vi "Main.vi"(11 "Module Admin":refnum<class "Delacor_lib_QMH_Module Admin.lvclass">) -> ()   [LabVIEW 2024, in "DAQ.lvlib"]
doc: "This template is based off of the Queued Message Handler design pattern and the Queued Message Handler project template that ships with LabVIEW.\n\nThe main difference is that the queue is private to this module and communication between modules is performed via Broadcast and Request events.\n\nRequest events are wrapped in public API methods and are handled in the Event Handling Loop (EHL) of this VI. Any module can register for Broadcast events sent by this module. The EHL generates messages based on user interface actions.\n\nThe Message Handling Loop (MHL) processes messages generated by the EHL, or by other messages. The messages are string values, so new messages can be added easily to the Message Cases case structure in the MHL. Each message cluster can also provide an optional value for Message Data, which is a variant that can be converted to whatever message-specific data is required.\n_____\nBased on DQMH Project Template 7.0.1.1316."
uses:
  DAQ.lvlib
  <vilib>/Delacor/Delacor QMH/Libraries/Module Admin_class/Delacor_lib_QMH_Module Admin.lvclass
  Module Data--cluster.ctl
  DAQ Config.ctl
  <vilib>/Delacor/Delacor QMH/Libraries/Message Queue_class/Delacor_lib_QMH_Message Queue.lvclass/Delacor_lib_QMH_Message Queue.ctl
  Stop Argument--cluster.ctl
  <vilib>/Delacor/Delacor QMH/Libraries/Module Admin_class/Delacor_lib_QMH_Module Admin.lvclass/Delacor_lib_QMH_Module Admin.ctl
  Configure Acquisition Argument--cluster.ctl
  Start Acquisition Argument--cluster.ctl
  Acquire Argument--cluster.ctl
  Stop Acquisition Argument--cluster.ctl
  <vilib>/Utility/miscctls.llb/LVPointTypeDef.ctl
  <vilib>/Delacor/Delacor QMH/Libraries/Message Queue_class/Delacor_lib_QMH_Enqueue Message (Single).vi
  <vilib>/Delacor/Delacor QMH/Libraries/Module Admin_class/Delacor_lib_QMH_Get External Launch.vi
  <vilib>/DAQmx/create/channels.llb/DAQmx Create Channel (AI-Voltage-Basic).vi
  <vilib>/DAQmx/configure/timing.llb/DAQmx Timing (Sample Clock).vi
  <vilib>/DAQmx/miscellaneous.llb/DAQmx Fill In Error Info.vi
  <vilib>/Delacor/Delacor QMH/Libraries/Message Queue_class/Delacor_lib_QMH_Message Queue.lvclass
  <vilib>/DAQmx/read.llb/DAQmx Read (Analog 1D Wfm NChan NSamp).vi
panel:
  out "Waveform Chart":waveform(dbl)[](graph)
  out "error out":errorcluster
  out "Status":string
  in  "Simulate MHL Error":bool
  in  "Simulate EHL Error":bool
  # "DAQ Module"
  # "This Module runs without a UI"
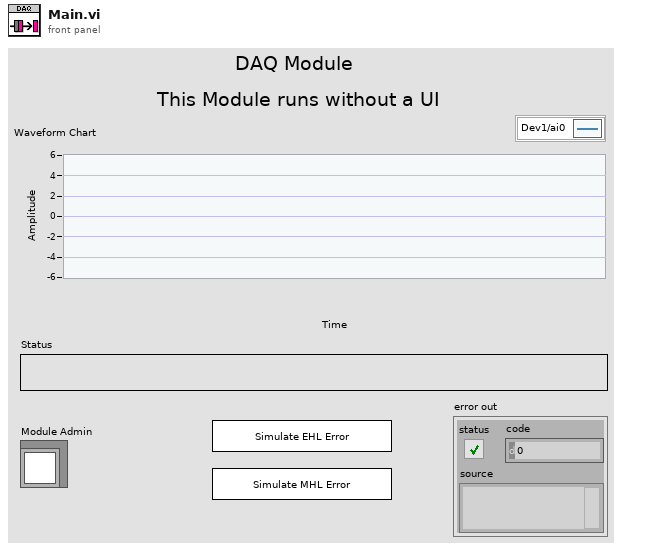
[diagram p1: front panel]
types:
  T1 = typedef "DAQ.lvlib/Request Events--cluster.ctl" = cluster{"Stop Module":refnum<user-event>, "Show Panel":refnum<user-event>, "Hide Panel":refnum<user-event>, "Get Module Execution Status":refnum<user-event>, "Show Diagram":refnum<user-event>, "Configure Acquisition":refnum<user-event>, "Start Acquisition":refnum<user-event>, "Private":cluster{"Acquire":refnum<user-event>}, "Stop Acquisition":refnum<user-event>}
  T2 = typedef "DAQ.lvlib/Module Data--cluster.ctl" = cluster{"Status":string, "DAQ Config":T3, "DAQmx task":refnum<k21>, "Stop Acquisition?":bool}
  T3 = typedef "DAQ.lvlib/DAQ Config.ctl" = cluster{"DAQmx Channel":tag, "Samplerate":dbl, "# Samples":i32}
  T4 = enum32{"invalid lock state", "Not Locked", "Locked (No Password)", "Password-protected"}
  T5 = typedef "DAQ.lvlib/Stop Argument--cluster.ctl" = cluster{"Origin":string, "Exit via Stop Module Req?":bool, "Wait for Module to stop?":bool}
  T6 = typedef "DAQ.lvlib/Configure Acquisition Argument--cluster.ctl" = cluster{"DAQ Config":T3}
  T7 = typedef "DAQ.lvlib/Start Acquisition Argument--cluster.ctl" = cluster{"Boolean":bool}
  T8 = typedef "DAQ.lvlib/Acquire Argument--cluster.ctl" = cluster{"Boolean":bool}
  T9 = typedef "DAQ.lvlib/Stop Acquisition Argument--cluster.ctl" = cluster{"Boolean":bool}
  T10 = typedef "LVPointTypeDef.ctl" = cluster{"Horizontal":i16, "Vertical":i16}
  T11 = enum32{"Invalid", "Standard", "Closed", "Hidden", "Minimized", "Maximized"}
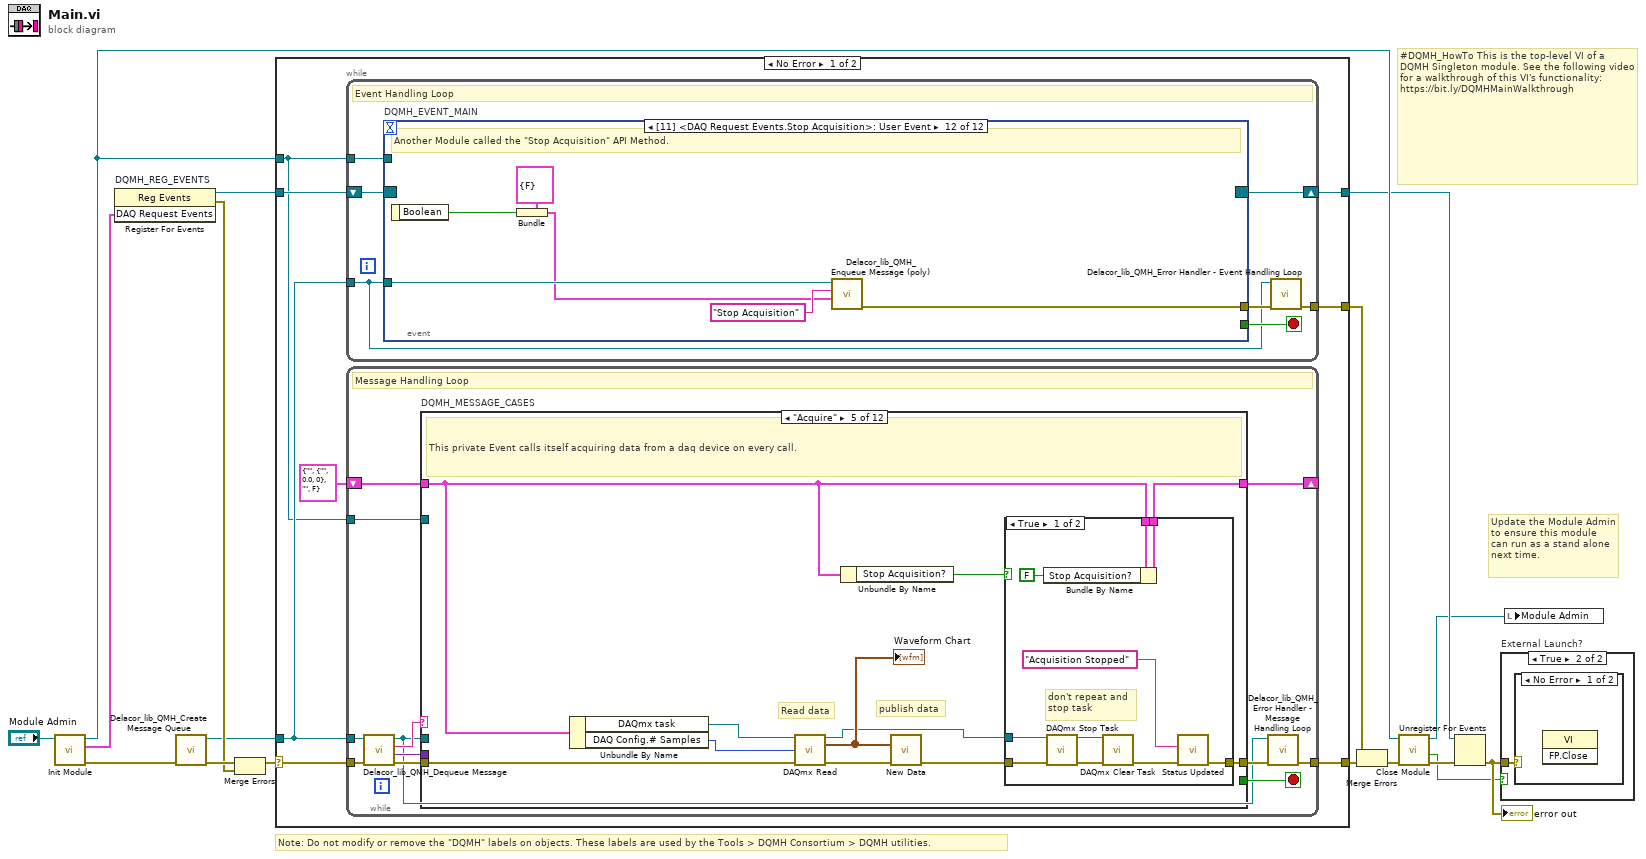
[diagram p0: block diagram]
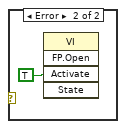
[diagram p3: hidden frame]
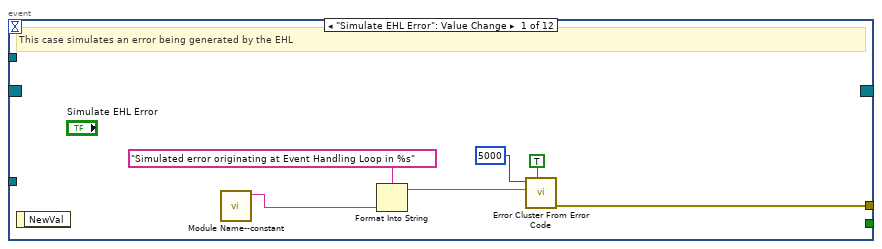
[diagram p4: hidden frame]
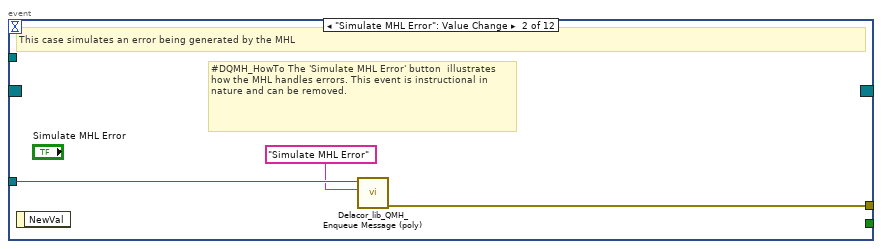
[diagram p5: hidden frame]
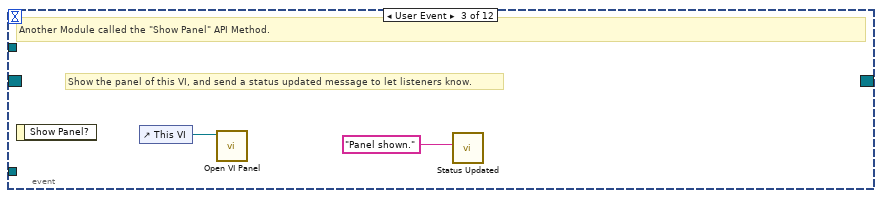
[diagram p6: hidden frame]
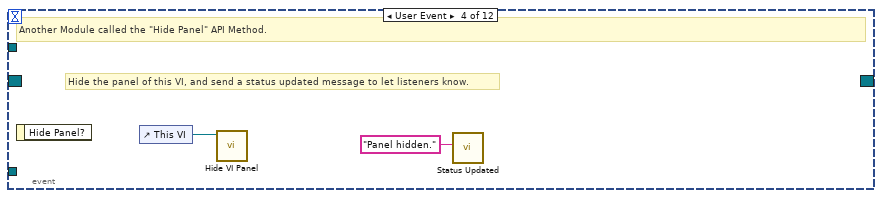
[diagram p7: hidden frame]
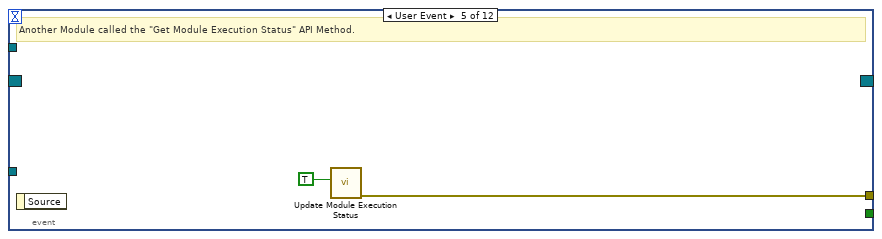
[diagram p8: hidden frame]
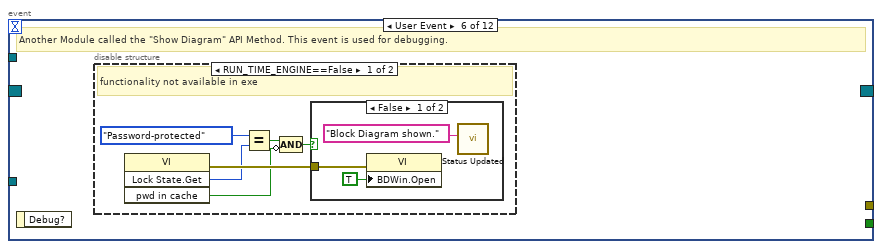
[diagram p9: hidden frame]
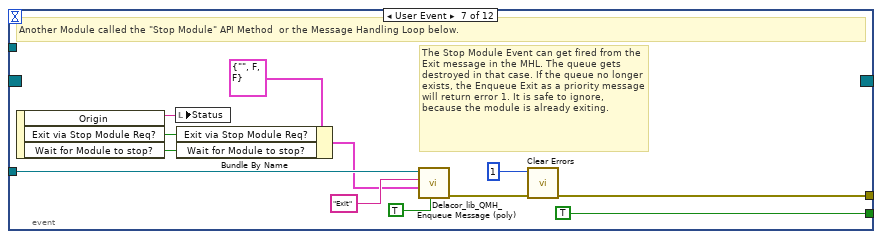
[diagram p12: hidden frame]
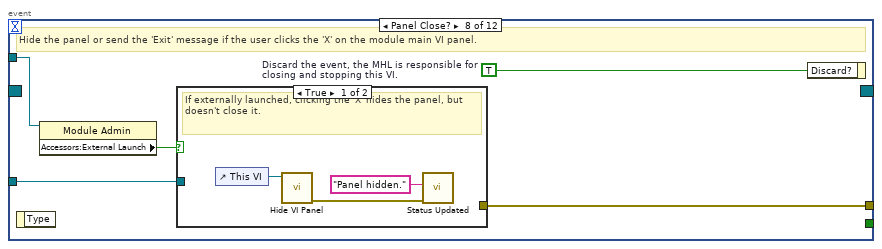
[diagram p13: hidden frame]
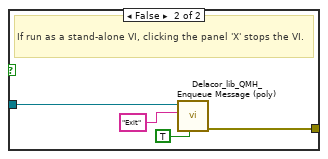
[diagram p14: hidden frame]
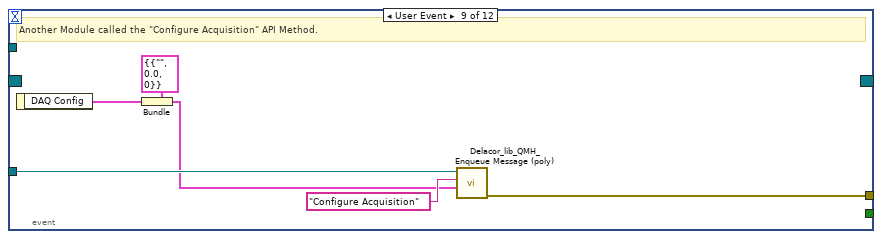
[diagram p15: hidden frame]
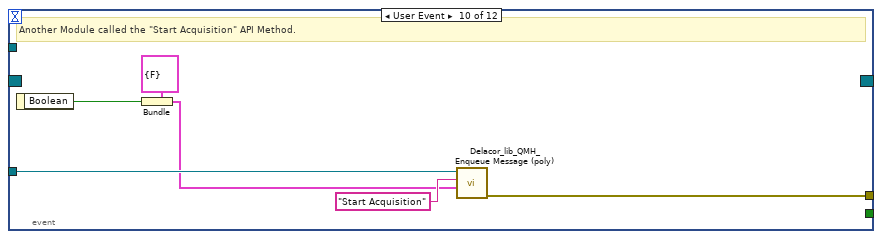
[diagram p16: hidden frame]
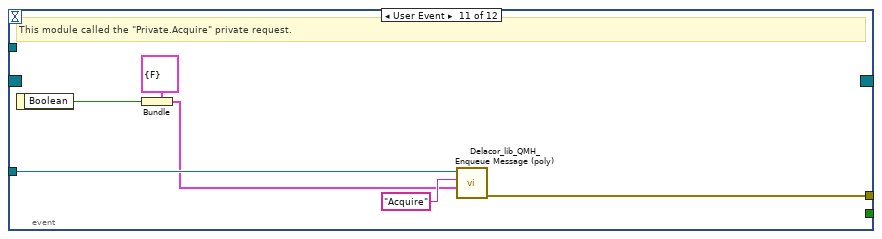
[diagram p17: hidden frame]
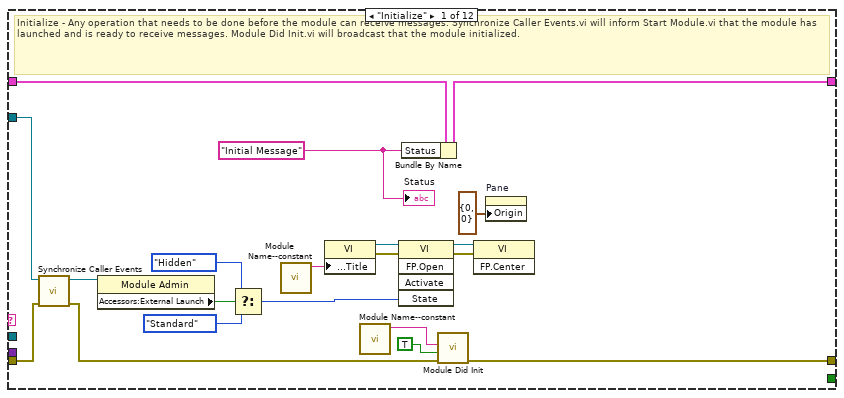
[diagram p18: hidden frame]
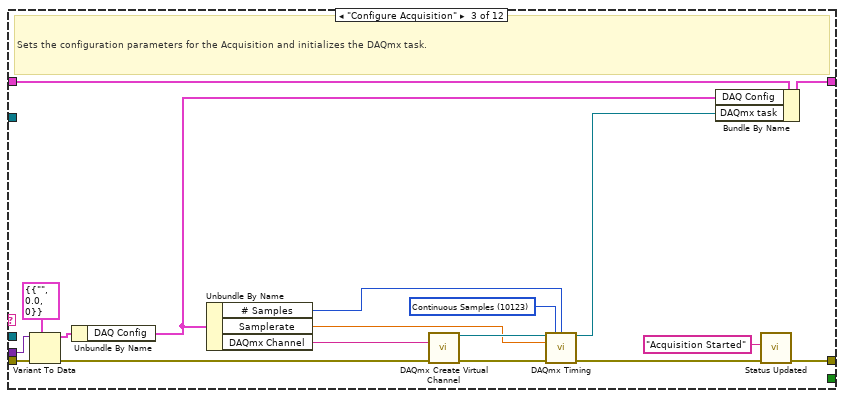
[diagram p20: hidden frame]
diagram:
  # "#DQMH_HowTo This is the top-level VI of a DQMH Singleton module. See the following video for a walkthrough of this VI's functionality: https://bit.ly/DQMHMainWalkthrough"
  # "Note: Do not modify or remove the \"DQMH\" labels on objects. These labels are used by the Tools > DQMH Consortium > DQMH utilities."
  # "Update the Module Admin to ensure this module can run as a stand alone next time."
  n1 = call "Init Module.vi"("Singleton Module Admin in"="Module Admin") -> ("error out"=w16:errorcluster, "DAQ Request Events"=w5:T1, "Singleton Module Admin out"=w8:refnum<class "Delacor_lib_QMH_Module Admin.lvclass">)  [unwired: 8 in]
  n2 = register-events "DQMH_REG_EVENTS"(w5) -> (reference out=w6:refnum<event-registration>, error out=w9:errorcluster)  [unwired: 2 in]
  n3 = call <vilib>:"Delacor_lib_QMH_Create Message Queue.vi"("error in"=w16) -> ("error out"=w11:errorcluster, "Message Queue"=w4:refnum<class "Delacor_lib_QMH_Message Queue.lvclass">)  [unwired: 9 in]
  n4 = Merge Errors(w11, w9) -> (w10:errorcluster)
  n5 = case shown="No Error" w10 {
    selector: w10 -> [w23 w253]
    tunnel: [w25 w252] -> w17
    tunnel: [w22 w251] -> w7
    tunnel: w6 -> [w20 w251]
    tunnel: w4 -> [w19 w246]
    tunnel: [w24 _] -> w14
    tunnel: w8 -> [w18 w247]
    frame No Error {
      n6 = while {
        tunnel: w19 -> [w26]
        shift-right: [w29] -> w22
        shift-left: w20 -> [w30]
        tunnel: [w31] -> w24
        tunnel: w18 -> [w27]
        stop <- w28 stop-if-true
        # "Event Handling Loop"
        n7 = event "DQMH_EVENT_MAIN" shown="[11] <DAQ Request Events.Stop Acquisition>: User Event" {
          selector: w30 -> [_ _ _ _ _ _ _ _ _ _ _ _]
          dyn-events: [_ _ _ _ _ _ _ _ _ _ _ _] -> w29
          timeout: _ -> [_ _ _ _ _ _ _ _ _ _ _ _]
          tunnel: [_ _ _ _ _ _ TRUE ("Discard?") _ _ _ _ _] -> w28
          tunnel: w26 -> [_ w40 _ _ _ _ w64 w71 w86 w92 w98 w104]
          tunnel: [w38 w41 _ _ w47 _ w67 w73 w81 w87 w93 w99] -> w32
          tunnel: w27 -> [_ _ _ _ _ _ _ w70 _ _ _ _]
          event "Simulate EHL Error": Value Change {
            # "This case simulates an error being generated by the EHL"
            n8 = event-data() -> ()  [unwired: 1 in, 1 out]
            n9 = call "Module Name--constant.vi"() -> ("Module Name"=w35:string)  [unwired: 11 in]
            n10 = Format Into String(format string="Simulated error originating at Event Handling Loop in %s", w35) -> (resulting string=w36:string)  [unwired: 2 in, 1 out]
            n11 = call <vilib>:"Error Cluster From Error Code.vi"("show call chain? (False)"=TRUE, "error message (\"\")"=w36, "error code (0)"=5000) -> ("error out"=w38:errorcluster)  [unwired: 6 in]
          }
          event "Simulate MHL Error": Value Change {
            # "#DQMH_HowTo The 'Simulate MHL Error' button  illustrates how the MHL handles errors. This event is instructional in nature and can be removed."
            # "This case simulates an error being generated by the MHL"
            n12 = event-data() -> ()  [unwired: 1 in, 1 out]
            n13 = call-poly <vilib>:"Delacor_lib_QMH_Enqueue Message (poly).vi"("Message"="Simulate MHL Error", "Message Queue in"=w40) -> ("error out"=w41:errorcluster)  [unwired: 8 in, 1 out]
          }
          event User Event {
            # "Show the panel of this VI, and send a status updated message to let listeners know."
            # "Another Module called the \"Show Panel\" API Method."
            n14 = event-data() -> ()  [unwired: 1 in, 1 out]
            n15 = control-ref of="This VI"() -> (w43:refnum<vi>)
            n16 = call "Open VI Panel.vi"("VI"=w43) -> ()  [unwired: 10 in, 1 out]
            n17 = call "Status Updated.vi"("Status"="Panel shown." ("format string")) -> ()  [unwired: 10 in, 1 out]
          }
          event User Event {
            # "Hide the panel of this VI, and send a status updated message to let listeners know."
            # "Another Module called the \"Hide Panel\" API Method."
            n18 = event-data() -> ()  [unwired: 1 in, 1 out]
            n19 = control-ref of="This VI"() -> (w45:refnum<vi>)
            n20 = call "Hide VI Panel.vi"("VI"=w45) -> ()  [unwired: 10 in, 1 out]
            n21 = call "Status Updated.vi"("Status"="Panel hidden." ("format string")) -> ()  [unwired: 10 in, 1 out]
          }
          event User Event {
            # "Another Module called the \"Get Module Execution Status\" API Method."
            n22 = event-data() -> ()  [unwired: 1 in, 1 out]
            n23 = call "Update Module Execution Status.vi"("Running?"=TRUE) -> ("error out"=w47:errorcluster)  [unwired: 10 in]
          }
          event User Event {
            # "Another Module called the \"Show Diagram\" API Method. This event is used for debugging."
            n24 = event-data() -> ()  [unwired: 1 in, 1 out]
            n25 = disable-structure shown="RUN_TIME_ENGINE==False" {
              frame condition #0 (active) {
                # "functionality not available in exe"
                n26 = invoke on="Invoke Node" class="VI" method="Lock State.Get"() -> (error out=w53:errorcluster, "Get Lock State"=w52:T4, "pwd in cache"=w49:bool)  [unwired: 4 in, 1 out]
                n27 = Equal?(x=T4."Password-protected", y=w52) -> (x = y?=w50:bool)
                n28 = Compound Arithmetic op=AND(w50, invert w49) -> (w48:bool)
                n29 = case shown="False" w48 {
                  tunnel: w53 -> [w56 _]
                  frame False {
                    n30 = property on="Property Node" class="VI"(error in=w56, "BDWin.Open"=TRUE ("Block Diagram Window:Open")) -> ()  [unwired: 1 in, 2 out]
                    n31 = call "Status Updated.vi"("Status"="Block Diagram shown." ("format string")) -> ()  [unwired: 10 in, 1 out]
                  }
                  frame True {
                    # "Password-protected VI, and the password is not in the cache. Do not show the diagram."
                  }
                }
              }
              frame condition #1 {
              }
            }
          }
          event User Event {
            # "The Stop Module Event can get fired from the Exit message in the MHL. The queue gets destroyed in that case. If the queue no longer exists, the Enqueue Exit as a priority message will return error 1. It is safe to ignore, because the module is already exiting."
            # "Another Module called the \"Stop Module\" API Method  or the Message Handling Loop below."
            n32 = event-data() -> ("Origin"=w63:string, "Exit via Stop Module Req?"=w59:bool, "Wait for Module to stop?"=w58:bool)  [unwired: 1 in]
            n33 = local write "Status"(w63) -> ()
            n34 = Bundle By Name(cluster=T5 {"Origin"="", "Exit via Stop Module Req?"=FALSE, "Wait for Module to stop?"=FALSE} ("Stop Argument"), "Exit via Stop Module Req?"=w59, "Wait for Module to stop?"=w58) -> (w57:T5)
            n35 = call-poly <vilib>:"Delacor_lib_QMH_Enqueue Message (poly).vi"("Priority Message? (F)"=TRUE, "Message Data"=w57, "Message"="Exit", "Message Queue in"=w64) -> ("error out"=w68:errorcluster)  [unwired: 6 in, 1 out]
            n36 = call <vilib>:"Clear Errors.vi"("error in (no error)"=w68, "specific error code to clear (0: all)"=1) -> ("error out"=w67:errorcluster)  [unwired: 4 in, 1 out]
          }
          event Panel Close? {
            w72 = TRUE  # Discard the event, the MHL is responsible for closing and stopping this VI.
            # "Hide the panel or send the 'Exit' message if the user clicks the 'X' on the module main VI panel."
            n37 = event-data() -> ()  [unwired: 1 in, 1 out]
            n38 = property on="Property Node" class="Module Admin"(reference=w70) -> ("Accessors:External Launch"=w69:bool)  [unwired: 1 in, 2 out]
            n39 = case shown="True" w69 {
              tunnel: w71 -> [_ w79]
              tunnel: [_ w80] -> w73
              frame True {
                # "If externally launched, clicking the 'X' hides the panel, but doesn't close it."
                n40 = control-ref of="This VI"() -> (w76:refnum<vi>)
                n41 = call "Hide VI Panel.vi"("VI"=w76) -> ("error out"=w74:errorcluster)  [unwired: 10 in]
                n42 = call "Status Updated.vi"("error in"=w74, "Status"="Panel hidden." ("format string")) -> ()  [unwired: 9 in, 1 out]
              }
              frame False {
                # "If run as a stand-alone VI, clicking the panel 'X' stops the VI."
                n43 = call-poly <vilib>:"Delacor_lib_QMH_Enqueue Message (poly).vi"("Priority Message? (F)"=TRUE, "Message"="Exit", "Message Queue in"=w79) -> ("error out"=w80:errorcluster)  [unwired: 7 in, 1 out]
              }
            }
            n44 = event-data ("Event Filter Node")("Discard?"=w72) -> ()  [unwired: 1 in, 1 out]
          }
          event User Event {
            # "Another Module called the \"Configure Acquisition\" API Method."
            n45 = event-data() -> ("DAQ Config"=w82:T3)  [unwired: 1 in]
            n46 = Bundle(cluster=T6 {"DAQ Config"={"DAQmx Channel"="", "Samplerate"=0.0, "# Samples"=0}} ("Configure Acquisition Argument"), "DAQ Config"=w82) -> (w83:T6)
            n47 = call-poly <vilib>:"Delacor_lib_QMH_Enqueue Message (poly).vi"("Message Data"=w83, "Message"="Configure Acquisition", "Message Queue in"=w86) -> ("error out"=w81:errorcluster)  [unwired: 7 in, 1 out]
          }
          event User Event {
            # "Another Module called the \"Start Acquisition\" API Method."
            n48 = event-data() -> ("Boolean"=w88:bool)  [unwired: 1 in]
            n49 = Bundle(cluster=T7 {"Boolean"=FALSE} ("Start Acquisition Argument"), "Boolean"=w88) -> (w89:T7)
            n50 = call-poly <vilib>:"Delacor_lib_QMH_Enqueue Message (poly).vi"("Message Data"=w89, "Message"="Start Acquisition", "Message Queue in"=w92) -> ("error out"=w87:errorcluster)  [unwired: 7 in, 1 out]
          }
          event User Event {
            # "This module called the \"Private.Acquire\" private request."
            n51 = event-data() -> ("Boolean"=w94:bool)  [unwired: 1 in]
            n52 = Bundle(cluster=T8 {"Boolean"=FALSE} ("Acquire Argument"), "Boolean"=w94) -> (w95:T8)
            n53 = call-poly <vilib>:"Delacor_lib_QMH_Enqueue Message (poly).vi"("Message Data"=w95, "Message"="Acquire", "Message Queue in"=w98) -> ("error out"=w93:errorcluster)  [unwired: 7 in, 1 out]
          }
          event User Event {
            # "Another Module called the \"Stop Acquisition\" API Method."
            n54 = event-data() -> ("Boolean"=w100:bool)  [unwired: 1 in]
            n55 = Bundle(cluster=T9 {"Boolean"=FALSE} ("Stop Acquisition Argument"), "Boolean"=w100) -> (w101:T9)
            n56 = call-poly <vilib>:"Delacor_lib_QMH_Enqueue Message (poly).vi"("Message Data"=w101, "Message"="Stop Acquisition", "Message Queue in"=w104) -> ("error out"=w99:errorcluster)  [unwired: 7 in, 1 out]
          }
        }
        n57 = call-dynamic "Delacor_lib_QMH_Error Handler - Event Handling Loop.vi"("error in"=w32, "Message Queue in"=w26) -> ("dup error in"=w31:errorcluster)  [unwired: 8 in, 1 out]
      }
      n58 = while {
        tunnel: w19 -> [w105]
        shift-right: [w113] -> _
        shift-left: T2 {"Status"="", "DAQ Config"={"DAQmx Channel"="", "Samplerate"=0.0, "# Samples"=0}, "DAQmx task"="", "Stop Acquisition?"=FALSE} ("Data Cluster") -> [w114]
        tunnel: w23 -> [w116]
        tunnel: [w108] -> w25
        tunnel: w18 -> [w109]
        stop <- w112 stop-if-true
        # "Message Handling Loop"
        n59 = call-dynamic "Delacor_lib_QMH_Dequeue Message.vi"("error in"=w116, "Message Queue in"=w105) -> ("error out"=w115:errorcluster, "Message Data"=w110:variant, "Message"=w111:string, "Message Queue out"=w106:refnum<class "Delacor_lib_QMH_Message Queue.lvclass">)  [unwired: 6 in]
        n60 = case "DQMH_MESSAGE_CASES" shown="\"Acquire\"" w111 {
          selector: w111 -> [_ _ _ _ _ _ _ _ _ _ _ w241]
          tunnel: w106 -> [_ _ _ _ _ _ _ _ _ w207 w229 _]
          tunnel: w115 -> [w134 w138 w156 w160 w171 w188 w192 w194 w203 w214 w235 w244]
          tunnel: [w132 w138 w140 w159 w172 w188 w191 w194 w202 w210 w230 w245] -> w107
          tunnel: w114 -> [w123 w137 w155 w161 w165 w189 w190 w193 w200 w209 w228 w242]
          tunnel: [w122 w137 w150 w161 w166 w187 w190 w193 w200 w209 w228 w242] -> w113
          tunnel: [_ _ _ _ _ _ _ _ _ _ w227 _] -> w112
          tunnel: w110 -> [_ _ w153 _ _ _ _ _ _ w208 w226 _]
          tunnel: w109 -> [w124 _ _ _ _ _ _ _ _ w206 w221 _]
          frame "Initialize" {
            w118 = "Initial Message" ("Initial Message")
            # "Initialize - Any operation that needs to be done before the module can receive messages. Synchronize Caller Events.vi will inform Start Module.vi that the module has launched and is ready to receive messages. Module Did Init.vi will broadcast that the module initialized."
            n61 = call "Synchronize Caller Events.vi"("error in"=w134, "Singleton Module Admin in"=w124) -> ("error out"=w133:errorcluster, "Singleton Module Admin out"=w119:refnum<class "Delacor_lib_QMH_Module Admin.lvclass">)  [unwired: 8 in]
            n62 = property on="Property Node" class="Module Admin"(reference=w119) -> ("Accessors:External Launch"=w128:bool)  [unwired: 1 in, 2 out]
            n63 = Select(t=T11."Hidden" ("State"), s=w128, f=T11."Standard" ("State")) -> (s? t:f=w125:T11)
            n64 = call "Module Name--constant.vi"() -> ("Module Name"=w131:string)  [unwired: 11 in]
            n65 = property on="Property Node" class="VI"("Front Panel.Title"=w131) -> (reference out=w130:refnum<vi>, error out=w136:errorcluster)  [unwired: 2 in]
            n66 = call "Module Name--constant.vi"() -> ("Module Name"=w120:string)  [unwired: 11 in]
            n67 = invoke on="Invoke Node" class="VI" method="FP.Open"(reference=w130, error in=w136, "State"=w125) -> (reference out=w129:refnum<vi>, error out=w135:errorcluster)  [unwired: 2 in, 3 out]
            n68 = Bundle By Name(cluster=w123, "Status"=w118) -> (w122:T2)
            n69 = call "Module Did Init.vi"("error in"=w133, "Initialized?"=TRUE, "Origin"=w120) -> ("error out"=w132:errorcluster)  [unwired: 8 in]
            n70 = invoke on="Invoke Node" class="VI" method="FP.Center"(reference=w129, error in=w135) -> ()  [unwired: 1 in, 3 out]
            n71 = property on="Pane" class="Pane"("Origin"=T10 {"Horizontal"=0, "Vertical"=0}) -> ()  [unwired: 2 in, 2 out]
            "Status" <- w118
          }
          frame "---Module Specific---" {
            # "Separator -- The following cases handle messages specific to this Module."
          }
          frame "Configure Acquisition" {
            w143 = 10123 items=["Finite Samples"=10178, "Continuous Samples"=10123, "Hardware Timed Single Point"=12522] ("sample mode")
            # "Sets the configuration parameters for the Acquisition and initializes the DAQmx task."
            n72 = Variant To Data(error in=w156, type=T6 {"DAQ Config"={"DAQmx Channel"="", "Samplerate"=0.0, "# Samples"=0}} ("Configure Acquisition Argument"), Variant=w153) -> (data=w151:T6, error out=w154:errorcluster)
            n73 = Unbundle By Name(w151) -> ("DAQ Config"=w148:T3)
            n74 = Unbundle By Name(w148) -> ("# Samples"=w142:i32, "Samplerate"=w144:dbl, "DAQmx Channel"=w147:tag)
            n75 = call-poly <vilib>:"DAQmx Create Virtual Channel.vi"("physical channels"=w147, "error in"=w154) -> ("task out"=w145:refnum<k21>, "error out"=w149:errorcluster)  [unwired: 12 in]
            n76 = call-poly <vilib>:"DAQmx Timing.vi"("task/channels in"=w145, "sample mode"=w143, "samples per channel"=w142, "rate"=w144, "error in"=w149) -> ("task out"=w141:refnum<k21>, "error out"=w146:errorcluster)  [unwired: 9 in]
            n77 = Bundle By Name(cluster=w155, "DAQ Config"=w148, "DAQmx task"=w141) -> (w150:T2)
            n78 = call "Status Updated.vi"("error in"=w146, "Status"="Acquisition Started") -> ("error out"=w140:errorcluster)  [unwired: 9 in]
          }
          frame "Start Acquisition" {
            # "Starts the DAQ Acquisition, the module will continue running until \"Stop Acquisition\" is called."
            n79 = call "Status Updated.vi"("error in"=w160, "Status"="Acquisition Started") -> ("error out"=w158:errorcluster)  [unwired: 9 in]
            n80 = call "Acquire.vi"("error in"=w158) -> ("error out"=w159:errorcluster)  [unwired: 10 in]
          }
          frame "Acquire" {
            # "publish data"
            # "Read data"
            # "This private Event calls itself acquiring data from a daq device on every call."
            n81 = Unbundle By Name(w165) -> ("DAQmx task"=w168:refnum<k21>, "DAQ Config.# Samples"=w167:i32)
            n82 = call-poly <vilib>:"DAQmx Read.vi"("task/channels in"=w168, "number of samples per channel"=w167, "error in"=w171) -> ("task out"=w162:refnum<k21>, "data"=w163:waveform(dbl)[], "error out"=w169:errorcluster)  [unwired: 10 in]
            "Waveform Chart" <- w163
            n83 = Unbundle By Name(w165) -> ("Stop Acquisition?"=w164:bool)
            n84 = call "New Data.vi"("error in"=w169, "Data"=w163) -> ("error out"=w170:errorcluster)  [unwired: 9 in]
            n85 = case shown="True" w164 {
              tunnel: [w174 w185] -> w172
              tunnel: w170 -> [w182 w184]
              tunnel: w165 -> [w181 w183]
              tunnel: [w180 w183] -> w166
              tunnel: w162 -> [w175 _]
              frame True {
                # "don't repeat and\nstop task"
                n86 = Bundle By Name(cluster=w181, "Stop Acquisition?"=FALSE) -> (w180:T2)
                n87 = call <vilib>:"DAQmx Stop Task.vi"("task/channels in"=w175, "error in"=w182) -> ("task out"=w176:refnum<k21>, "error out"=w178:errorcluster)  [unwired: 12 in]
                n88 = call <vilib>:"DAQmx Clear Task.vi"("task in"=w176, "error in"=w178) -> ("error out"=w177:errorcluster)  [unwired: 13 in]
                n89 = call "Status Updated.vi"("error in"=w177, "Status"="Acquisition Stopped") -> ("error out"=w174:errorcluster)  [unwired: 9 in]
              }
              frame False {
                # "Repeat"
                n90 = call "Acquire.vi"("error in"=w184) -> ("error out"=w185:errorcluster)  [unwired: 10 in]
              }
            }
          }
          frame "Stop Acquisition" {
            # "Stops the continuous Acquisition."
            n91 = Bundle By Name(cluster=w189, "Stop Acquisition?"=TRUE) -> (w187:T2)
          }
          frame "---Copy This Frame---" {
            # "Duplicate this frame when creating new messages.  Change this comment in the duplicated frame to describe this message."
            n92 = Merge Errors(w192) -> (w191:errorcluster)
          }
          frame "---Exit and Error Handling---" {
            # "Separator - The following cases handle errors and exit messages."
          }
          frame "Simulate MHL Error" {
            # "#DQMH_HowTo The 'Simulate MHL Error' button  illustrates how the MHL handles errors. This event is instructional in nature and can be removed."
            # "Simulate an error occurring at the MHL"
            n93 = call "Module Name--constant.vi"() -> ("Module Name"=w196:string)  [unwired: 11 in]
            n94 = Format Into String(format string="Simulated error originating at Message Handling Loop in %s", w196) -> (resulting string=w197:string)  [unwired: 2 in, 1 out]
            n95 = call <vilib>:"Error Cluster From Error Code.vi"("show call chain? (False)"=TRUE, "error message (\"\")"=w197, "error code (0)"=5001) -> ("error out"=w201:errorcluster)  [unwired: 6 in]
            n96 = Merge Errors(w203, w201) -> (w202:errorcluster)
          }
          frame "Error" {
            # "#CodeRecommended - If the module is running in standalone mode (External Launch = FALSE), this code will pop up an error dialog and call the 'Exit' message if an error occurs. Add more fine-grained error management here."
            # "Error - Check the error message data and respond accordingly. This message is sent by the \"Error Handler\" VIs at the end of each loop in this application."
            n97 = property on="Property Node" class="Module Admin"(reference=w206) -> ("Accessors:External Launch"=w205:bool)  [unwired: 1 in, 2 out]
            n98 = Variant To Data(error in=w214, type=errorcluster {"status"=FALSE, "code"=0, "source"=""} ("error constant"), Variant=w208) -> (data=w204:errorcluster, error out=w212:errorcluster)
            n99 = local write "error out"(w204) -> ()
            n100 = call "Error Reported.vi"("Error"=w204) -> ()  [unwired: 10 in, 1 out]
            n101 = case shown="False" w205 {
              tunnel: [w219 _] -> w211
              tunnel: w207 -> [w217 _]
              tunnel: w204 -> [w218 _]
              frame False {
                n102 = disable-structure shown="Default" {
                  disable-tunnel: w218 -> [w220 _]
                  frame condition #0 (active) {
                    # "If the module is running standalone, then pop up an error dialog and call the \"Exit\" message."
                    n103 = call <vilib>:"Simple Error Handler.vi"("error in (no error)"=w220) -> ()  [unwired: 4 in, 5 out]
                  }
                  frame condition #1 {
                    # "To prevent the Simple Error Handler VI from being loaded (e.g. when deploying to a Real-Time target), add the Conditional Disable Symbol \"DQMH_Disable_SEH\" to your project and set it to TRUE."
                  }
                }
                n104 = call-poly <vilib>:"Delacor_lib_QMH_Enqueue Message (poly).vi"("Priority Message? (F)"=TRUE, "Message"="Exit", "Message Queue in"=w217) -> ("error out"=w219:errorcluster)  [unwired: 7 in, 1 out]
              }
              frame True {
                # "If the module was launched externally, calling the Error Reported broadcast VI is the only action performed by the \"Error\" message. The module's caller can then process the error appropriately."
              }
            }
            n105 = Merge Errors(w212, w211) -> (w210:errorcluster)
          }
          frame "Exit" {
            w225 = 91  # 91: not all Exit messages will have an argument
            w227 = TRUE  # Stop the VI
            # "Release the message queue reference"
            # "#CodeNeeded - Add any required cleanup code here."
            # "Exit - Exit the application."
            n106 = Variant To Data(error in=w235, type=T5 {"Origin"="", "Exit via Stop Module Req?"=FALSE, "Wait for Module to stop?"=FALSE} ("Stop Argument"), Variant=w226) -> (data=w223:T5, error out=w232:errorcluster)
            n107 = call <vilib>:"Clear Errors.vi"("error in (no error)"=w232, "specific error code to clear (0: all)"=w225) -> ("error out"=w234:errorcluster)  [unwired: 4 in, 1 out]
            n108 = control-ref of="This VI"() -> (w222:refnum<vi>)
            n109 = call-dynamic "Delacor_lib_QMH_Release Message Queue.vi"("error in"=w234, "Message Queue"=w229) -> ("error out"=w233:errorcluster)  [unwired: 9 in]
            n110 = call "Handle Exit.vi"("Stop Argument"=w223, "Admin in"=w221, "VI reference"=w222) -> ("error out"=w231:errorcluster)  [unwired: 7 in, 1 out]
            n111 = Merge Errors(w233, w231) -> (w230:errorcluster)
            n112 = call "Error Reported.vi"("Error"=w230) -> ()  [unwired: 10 in, 1 out]
          }
          frame Default {
            # "'Default' case only runs if there is a message that isn't defined in any of the other cases.  Output a programming error."
            n113 = call "Module Name--constant.vi"() -> ("Module Name"=w240:string)  [unwired: 11 in]
            n114 = Format Into String(format string="The invalid message string \"%s\" was received in the Message Handling Loop for module \"%s\".", w241, w240) -> (resulting string=w236:string)  [unwired: 2 in, 1 out]
            n115 = call <vilib>:"Error Cluster From Error Code.vi"("show call chain? (False)"=TRUE, "error message (\"\")"=w236, "error code (0)"=1) -> ("error out"=w243:errorcluster)  [unwired: 6 in]
            n116 = Merge Errors(w244, w243) -> (w245:errorcluster)
          }
        }
        n117 = call-dynamic "Delacor_lib_QMH_Error Handler - Message Handling Loop.vi"("error in"=w107, "Message Queue in"=w106) -> ("dup error in"=w108:errorcluster)  [unwired: 8 in, 1 out]
      }
    }
    frame Error {
      # "Synchronize Caller Events.vi will inform Start Module.vi that the module has launched and will let the code calling Start Module.vi register for broadcasts and would permit the caller receive the broadcast that an error occurred at launch time."
      n118 = call-dynamic "Delacor_lib_QMH_Release Message Queue.vi"("error in"=w253, "Message Queue"=w246) -> ("error out"=w252:errorcluster)  [unwired: 9 in]
      n119 = call "Synchronize Caller Events.vi"("Singleton Module Admin in"=w247) -> ("error out"=w254:errorcluster)  [unwired: 9 in, 1 out]
      n120 = call "Module Name--constant.vi"() -> ("Module Name"=w250:string)  [unwired: 11 in]
      n121 = Format Into String(format string="An error occurred during initialization. %s is no longer running.", w250) -> (resulting string=w248:string)  [unwired: 2 in, 1 out]
      n122 = Merge Errors(w252, w254) -> (w255:errorcluster)
      n123 = call "Error Reported.vi"("Additional Information"=w248, "Error"=w255) -> ()  [unwired: 9 in, 1 out]
    }
  }
  n124 = Merge Errors(w14, w17) -> (w13:errorcluster)
  n125 = call "Close Module.vi"("error in"=w13, "Module Admin in"=w8) -> ("error out"=w15:errorcluster, "External Launch"=w1:bool, "Module Admin out"=w2:refnum<class "Delacor_lib_QMH_Module Admin.lvclass">)  [unwired: 7 in]
  n126 = Unregister For Events(event registration refnum=w7, error in=w15) -> (error out=w12:errorcluster)
  "error out" <- w12
  n127 = case "External Launch?" shown="True" w1 {
    tunnel: w12 -> [_ w256]
    frame False {
    }
    frame True {
      n128 = case shown="No Error" w256 {
        frame No Error {
          n129 = invoke on="Invoke Node" class="VI" method="FP.Close"() -> ()  [unwired: 3 in, 3 out]
        }
        frame Error {
          n130 = invoke on="Invoke Node" class="VI" method="FP.Open"("Activate"=TRUE ("Activate?")) -> ()  [unwired: 4 in, 5 out]
        }
      }
    }
  }
  n131 = local write "Module Admin"(w2) -> ()
